vi "ConversionToUINT32.vi"(11 "uint byte tab":u8[](array[numeric])) -> (3 "Outcome":u32)   [LabVIEW 2015]
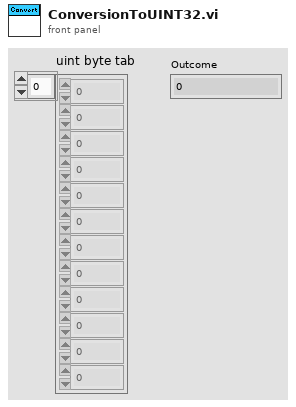
[diagram p1: front panel]
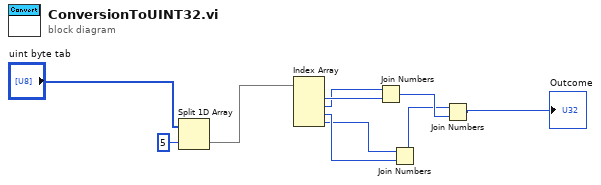
[diagram p0: block diagram]
diagram:
  n1 = Split 1D Array(array="uint byte tab", index=5) -> (second subarray=w8:u8[])  [unwired: 1 out]
  n2 = Index Array(array=w8) -> (element #1=w7:u8, element #2=w6:u8, element #3=w5:u8, element #4=w4:u8)  [unwired: 4 in]
  n3 = Join Numbers(hi=w6, lo=w7) -> ((hi.lo)=w3:u16)
  n4 = Join Numbers(hi=w4, lo=w5) -> ((hi.lo)=w2:u16)
  n5 = Join Numbers(hi=w2, lo=w3) -> ((hi.lo)=→"Outcome":u32)
